vi "LoadinTheStaticPictures_171213.vi"() -> (2 "background":picture, 3 "logo":picture)   [LabVIEW 2016]
uses:
  Globaltracker.vi
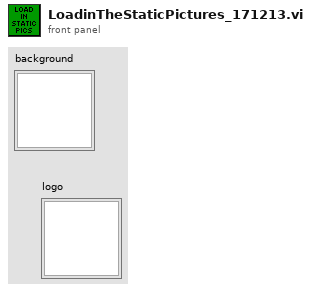
[diagram p1: front panel]
types:
  T1 = cluster{"Width":u16, "Style":enum32{"Solid", "Dash", "Dot", "DashDot", "DashDotDot"}}
  T2 = typedef "imagedata.ctl" = cluster{"image type":i32, "image depth":i32, "image":u8[], "mask":u8[], "colors":u32[], "Rectangle":cluster{"left":i16, "top":i16, "right":i16, "bottom":i16}}
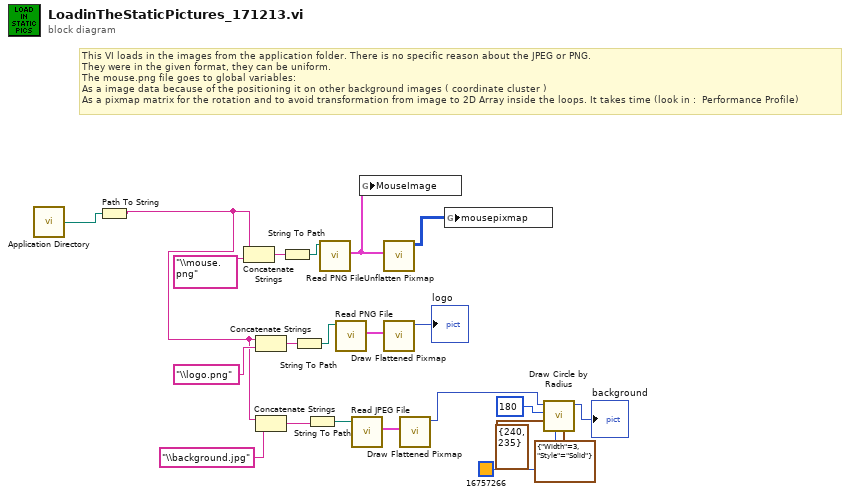
[diagram p0: block diagram]
diagram:
  # "This VI loads in the images from the application folder. There is no specific reason about the JPEG or PNG. \nThey were in the given format, they can be uniform.\nThe mouse.png file goes to global variables: \nAs a image data because of the positioning it on other background images ( coordinate cluster )\nAs a pixmap matrix for the rotation and to avoid transformation from image to 2D Array inside the loops. It takes time (look in :  Performance Profile)"
  n1 = call <vilib>:"Application Directory.vi"() -> ("Application Directory"=w8:path)
  n2 = Path To String(path=w8) -> (string=w7:string)
  n3 = Concatenate Strings(w7, "\\mouse.png" ("string")) -> (w21:string)
  n4 = Concatenate Strings(w7, "\\logo.png" ("string")) -> (w19:string)
  n5 = Concatenate Strings(w7, "\\background.jpg" ("string")) -> (w11:string)
  n6 = String To Path(string=w21) -> (path=w20:path)
  n7 = String To Path(string=w19) -> (path=w16:path)
  n8 = String To Path(string=w11) -> (path=w10:path)
  n9 = call <vilib>:"Read PNG File.vi"("path to PNG file"=w20) -> ("image data"=w18:T2)  [unwired: 8 in, 2 out]
  n10 = call <vilib>:"Read PNG File.vi"("path to PNG file"=w16) -> ("image data"=w15:T2)  [unwired: 8 in, 2 out]
  n11 = call <vilib>:"Read JPEG File.vi"("path to JPEG file"=w10) -> ("image data"=w9:T2)  [unwired: 8 in, 2 out]
  n12 = global write "Globaltracker.vi" "MouseImage"(w18) -> ()
  n13 = call <vilib>:"Unflatten Pixmap.vi"("image data"=w18) -> ("24-bit pixmap"=w17:u32[][])  [unwired: 4 in, 6 out]
  n14 = call <vilib>:"Draw Flattened Pixmap.vi"("image data"=w15) -> ("new picture"=→"logo":picture)  [unwired: 8 in]
  n15 = call <vilib>:"Draw Flattened Pixmap.vi"("image data"=w9) -> ("new picture"=w2:picture)  [unwired: 8 in]
  n16 = global write "Globaltracker.vi" "mousepixmap"(w17) -> ()
  n17 = call <vilib>:"Draw Circle by Radius.vi"("pen"=T1 {"Width"=3, "Style"=enum."Solid"}, "color(black)"=u32 16757266, "pixel center"=cluster{"horizontal":i16, "vertical":i16} {"horizontal"=240, "vertical"=235}, "radius"=i16 180, "picture"=w2) -> ("new picture"=→"background":picture)  [unwired: 6 in]
